vi "4x7segmentFunc.vi"(11 "Numeric Control":dbl format="%#_13g") -> (3 "?":T9)   [LabVIEW 2019]
uses:
  4x7 segment controls/top-segment-f.ctl
  4x7 segment controls/left-segment-f.ctl
  4x7 segment controls/rigt-segment-f.ctl
  4x7 segment controls/mid-segment-f.ctl
  4x7 segment controls/bottom-segment-f.ctl
  4x7 segment controls/decimal-f.ctl
  4x7 segment controls/kHz-f.ctl
  4x7 segment controls/Hz-f.ctl
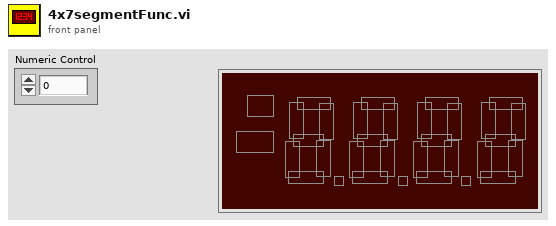
[diagram p1: front panel]
types:
  T1 = typedef "top-segment-f.ctl" = bool
  T2 = typedef "left-segment-f.ctl" = bool
  T3 = typedef "rigt-segment-f.ctl" = bool
  T4 = typedef "mid-segment-f.ctl" = bool
  T5 = typedef "bottom-segment-f.ctl" = bool
  T6 = typedef "decimal-f.ctl" = bool
  T7 = typedef "kHz-f.ctl" = bool
  T8 = typedef "Hz-f.ctl" = bool
  T9 = cluster{"1":cluster{"1":T1, "2":T2, "3":T3, "4":T4, "5":T2, "6":T3, "7":T5}, "2":cluster{"1":T1, "2":T2, "3":T3, "4":T4, "5":T2, "6":T3, "7":T5}, "3":cluster{"1":T1, "2":T2, "3":T3, "4":T4, "5":T2, "6":T3, "7":T5}, "4":cluster{"1":T1, "2":T2, "3":T3, "4":T4, "5":T2, "6":T3, "7":T5}, T6, T6, T6, T7, T8}
  T10 = cluster{"1":T1, "2":T2, "3":T3, "4":T4, "5":T2, "6":T3, "7":T5}
  T11 = cluster{"1":T1, "2":T2, "3":T3, "4":T4, "5":T2, "6":T3, "7":T5}[]
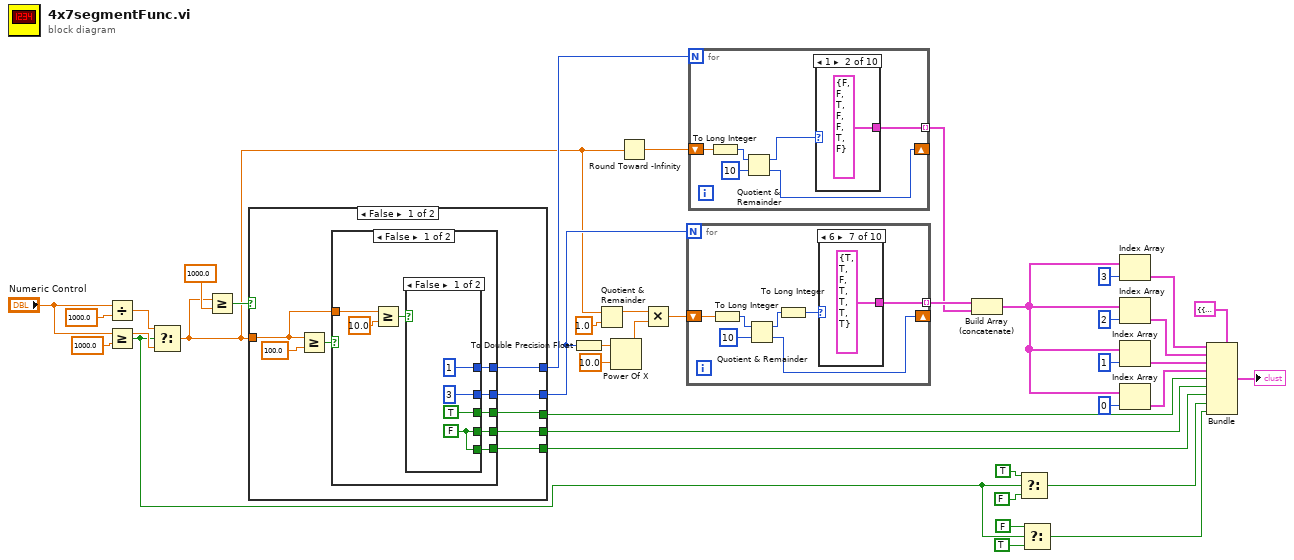
[diagram p0: block diagram]
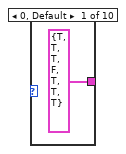
[diagram p2: hidden frame]
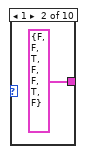
[diagram p3: hidden frame]
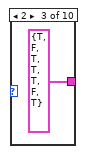
[diagram p4: hidden frame]
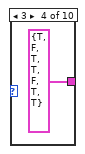
[diagram p5: hidden frame]
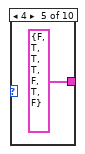
[diagram p6: hidden frame]
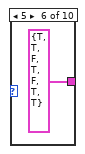
[diagram p7: hidden frame]
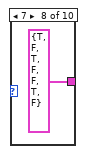
[diagram p8: hidden frame]
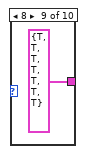
[diagram p9: hidden frame]
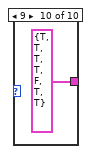
[diagram p10: hidden frame]
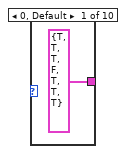
[diagram p11: hidden frame]
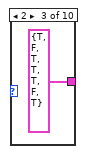
[diagram p12: hidden frame]
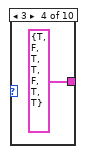
[diagram p13: hidden frame]
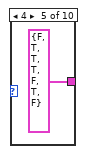
[diagram p14: hidden frame]
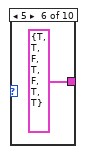
[diagram p15: hidden frame]
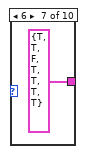
[diagram p16: hidden frame]
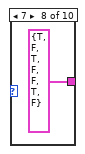
[diagram p17: hidden frame]
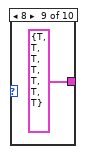
[diagram p18: hidden frame]
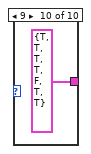
[diagram p19: hidden frame]
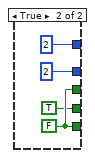
[diagram p20: hidden frame]
diagram:
  n1 = Divide(x="Numeric Control", y=1000.0) -> (x/y=w37:dbl)
  n2 = Greater Or Equal?(x="Numeric Control", y=1000.0) -> (x >= y?=w3:bool)
  n3 = Select(t=w37, s=w3, f="Numeric Control") -> (s? t:f=w10:dbl)
  n4 = Greater Or Equal?(x=w10, y=1000.0) -> (x >= y?=w13:bool)
  n5 = case shown="False" w13 {
    tunnel: [w43 w68] -> w28
    tunnel: [w42 w68] -> w27
    tunnel: [w44 w68] -> w26
    tunnel: w10 -> [w41 _]
    tunnel: [w45 4] -> w24
    tunnel: [w40 0] -> w17
    frame False {
      n6 = Greater Or Equal?(x=w41, y=100.0) -> (x >= y?=w46:bool)
      n7 = case shown="False" w46 {
        tunnel: [w49 3] -> w45
        tunnel: [w48 1] -> w40
        tunnel: [w52 T6 TRUE] -> w44
        tunnel: [w51 w64] -> w43
        tunnel: [w50 w64] -> w42
        tunnel: w41 -> [w55 _]
        frame False {
          n8 = Greater Or Equal?(x=w55, y=10.0) -> (x >= y?=w53:bool)
          n9 = case shown="False" w53 {
            tunnel: [w56 w63] -> w52
            tunnel: [T6 TRUE w63] -> w51
            tunnel: [w56 T6 TRUE] -> w50
            tunnel: [1 2] -> w49
            tunnel: [3 2] -> w48
            frame False {
              w56 = T6 FALSE
            }
            frame True {
              w63 = T6 FALSE
            }
          }
        }
        frame True {
          w64 = T6 FALSE
        }
      }
    }
    frame True {
      w68 = T6 FALSE
    }
  }
  n10 = To Double Precision Float(number=w17) -> (double precision float=w19:dbl)
  n11 = Quotient & Remainder(x=w10, y=1.0) -> (x-y*floor(x/y)=w22:dbl)  [unwired: 1 out]
  n12 = Power Of X(1:10.0 ("x"), 2:w19) -> (0:w21:dbl)
  n13 = Round Toward -Infinity(1:w10) -> (0:w11:dbl)
  n14 = Multiply(x=w22, y=w21) -> (x*y=w18:dbl)
  n15 = for {
    N: w17 -> [_]
    shift-right: [w77] -> _
    shift-left: w18 -> [w73]
    tunnel: [w74] -> w15 mode=indexing
    n16 = To Long Integer(number=w73) -> (32bit integer=w72:i32)
    n17 = Quotient & Remainder(x=w72, y=10) -> (x-y*floor(x/y)=w76:i32, floor(x/y)=w77:i32)
    n18 = To Long Integer(number=w76) -> (32bit integer=w75:i32)
    n19 = case shown="6" w75 {
      tunnel: [T10 {"1"=TRUE, "2"=TRUE, "3"=TRUE, "4"=FALSE, "5"=TRUE, "6"=TRUE, "7"=TRUE} ("1") T10 {"1"=FALSE, "2"=FALSE, "3"=TRUE, "4"=FALSE, "5"=FALSE, "6"=TRUE, "7"=FALSE} ("1") T10 {"1"=TRUE, "2"=FALSE, "3"=TRUE, "4"=TRUE, "5"=TRUE, "6"=FALSE, "7"=TRUE} ("1") T10 {"1"=TRUE, "2"=FALSE, "3"=TRUE, "4"=TRUE, "5"=FALSE, "6"=TRUE, "7"=TRUE} ("1") T10 {"1"=FALSE, "2"=TRUE, "3"=TRUE, "4"=TRUE, "5"=FALSE, "6"=TRUE, "7"=FALSE} ("1") T10 {"1"=TRUE, "2"=TRUE, "3"=FALSE, "4"=TRUE, "5"=FALSE, "6"=TRUE, "7"=TRUE} ("1") T10 {"1"=TRUE, "2"=TRUE, "3"=FALSE, "4"=TRUE, "5"=TRUE, "6"=TRUE, "7"=TRUE} ("1") T10 {"1"=TRUE, "2"=FALSE, "3"=TRUE, "4"=FALSE, "5"=FALSE, "6"=TRUE, "7"=FALSE} ("1") T10 {"1"=TRUE, "2"=TRUE, "3"=TRUE, "4"=TRUE, "5"=TRUE, "6"=TRUE, "7"=TRUE} ("1") T10 {"1"=TRUE, "2"=TRUE, "3"=TRUE, "4"=TRUE, "5"=FALSE, "6"=TRUE, "7"=TRUE} ("1")] -> w74
      frame 0, Default {
      }
      frame 1 {
      }
      frame 2 {
      }
      frame 3 {
      }
      frame 4 {
      }
      frame 5 {
      }
      frame 6 {
      }
      frame 7 {
      }
      frame 8 {
      }
      frame 9 {
      }
    }
  }
  n20 = for {
    N: w24 -> [_]
    shift-right: [w93] -> _
    shift-left: w11 -> [w91]
    tunnel: [w92] -> w14 mode=indexing
    n21 = To Long Integer(number=w91) -> (32bit integer=w90:i32)
    n22 = Quotient & Remainder(x=w90, y=10) -> (x-y*floor(x/y)=w89:i32, floor(x/y)=w93:i32)
    n23 = case shown="1" w89 {
      tunnel: [T10 {"1"=TRUE, "2"=TRUE, "3"=TRUE, "4"=FALSE, "5"=TRUE, "6"=TRUE, "7"=TRUE} ("1") T10 {"1"=FALSE, "2"=FALSE, "3"=TRUE, "4"=FALSE, "5"=FALSE, "6"=TRUE, "7"=FALSE} ("1") T10 {"1"=TRUE, "2"=FALSE, "3"=TRUE, "4"=TRUE, "5"=TRUE, "6"=FALSE, "7"=TRUE} ("1") T10 {"1"=TRUE, "2"=FALSE, "3"=TRUE, "4"=TRUE, "5"=FALSE, "6"=TRUE, "7"=TRUE} ("1") T10 {"1"=FALSE, "2"=TRUE, "3"=TRUE, "4"=TRUE, "5"=FALSE, "6"=TRUE, "7"=FALSE} ("1") T10 {"1"=TRUE, "2"=TRUE, "3"=FALSE, "4"=TRUE, "5"=FALSE, "6"=TRUE, "7"=TRUE} ("1") T10 {"1"=TRUE, "2"=TRUE, "3"=FALSE, "4"=TRUE, "5"=TRUE, "6"=TRUE, "7"=TRUE} ("1") T10 {"1"=TRUE, "2"=FALSE, "3"=TRUE, "4"=FALSE, "5"=FALSE, "6"=TRUE, "7"=FALSE} ("1") T10 {"1"=TRUE, "2"=TRUE, "3"=TRUE, "4"=TRUE, "5"=TRUE, "6"=TRUE, "7"=TRUE} ("1") T10 {"1"=TRUE, "2"=TRUE, "3"=TRUE, "4"=TRUE, "5"=FALSE, "6"=TRUE, "7"=TRUE} ("1")] -> w92
      frame 0, Default {
      }
      frame 1 {
      }
      frame 2 {
      }
      frame 3 {
      }
      frame 4 {
      }
      frame 5 {
      }
      frame 6 {
      }
      frame 7 {
      }
      frame 8 {
      }
      frame 9 {
      }
    }
  }
  n24 = Build Array (concatenate)(w15, w14) -> (w16:T11)
  n25 = Select(t=T7 TRUE, s=w3, f=T7 FALSE) -> (s? t:f=w2:T7)
  n26 = Select(t=T8 FALSE, s=w3, f=T8 TRUE) -> (s? t:f=w1:T8)
  n27 = Index Array(array=w16, index=3) -> (element=w32:T10)
  n28 = Index Array(array=w16, index=2) -> (element=w31:T10)
  n29 = Index Array(array=w16, index=1) -> (element=w30:T10)
  n30 = Index Array(array=w16, index=0) -> (element=w29:T10)
  n31 = Bundle(cluster=T9 {"1"={"1"=FALSE, "2"=FALSE, "3"=TRUE, "4"=FALSE, "5"=FALSE, "6"=TRUE, "7"=FALSE}, "2"={"1"=TRUE, "2"=TRUE, "3"=FALSE, "4"=TRUE, "5"=TRUE, "6"=TRUE, "7"=TRUE}, "3"={"1"=FALSE, "2"=TRUE, "3"=TRUE, "4"=TRUE, "5"=FALSE, "6"=TRUE, "7"=FALSE}, "4"={"1"=TRUE, "2"=TRUE, "3"=TRUE, "4"=FALSE, "5"=TRUE, "6"=TRUE, "7"=TRUE}, FALSE, FALSE, TRUE, FALSE, FALSE}, "1"=w32, "2"=w31, "3"=w30, "4"=w29, w28, w27, w26, w2, w1) -> (→"?":T9)
